vi "PLC版CODMn泵校准数据插入.vi"(0 "data":T1, 3 "错误输入（无错误）":errorcluster) -> (10 "错误输出":errorcluster)   [LabVIEW 2016, in "斯坦道CODMn.lvlib"]
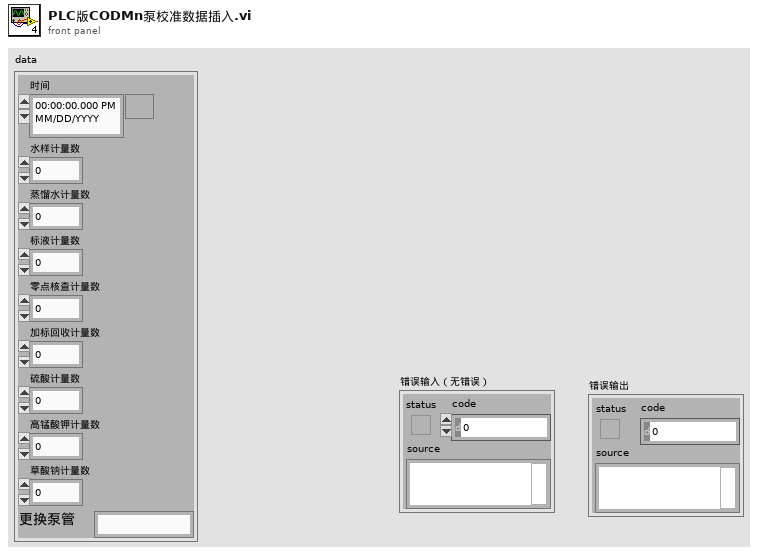
[diagram p1: front panel]
types:
  T1 = cluster{"时间":timestamp, "水样计量数":u16, "蒸馏水计量数":u16, "标液计量数":u16, "零点核查计量数":u16, "加标回收计量数":u16, "硫酸计量数":u16, "高锰酸钾计量数":u16, "草酸钠计量数":u16, "更换泵管":string}
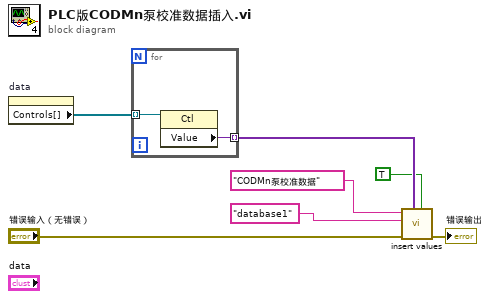
[diagram p0: block diagram]
diagram:
  n1 = property on="data" class="Clust (严格)"() -> ("Controls[]"=w7:refnum<vi>[])  [unwired: 2 in, 2 out]
  n2 = for {
    tunnel: w7 -> [w9] mode=indexing
    tunnel: [w8] -> w6 mode=indexing
    n3 = property class="Ctl"(reference=w9) -> ("Value"=w8:variant)  [unwired: 1 in, 2 out]
  }
  n4 = call "insert values.vi"("是否创建唯一键"=TRUE, "data"=w6, "错误输入（无错误）"="错误输入（无错误）", "database"="database1", "Tabe Name"="CODMn泵校准数据") -> ("错误输出"=→"错误输出":errorcluster)  [unwired: 6 in]
